vi "CRYCal Start Freq for TSR.vi"(6 "Hn":dbl=1.0, 8 "Over-samples Res.":dbl, 9 "sweep type":i32=1, 10 "FStart":dbl, 11 "Fs":dbl=2.0) -> (2 "Increment":dbl, 3 "Start Fs":dbl)   [LabVIEW 2013]
panel:
  out "x+y":dbl
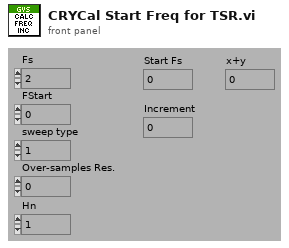
[diagram p1: front panel]
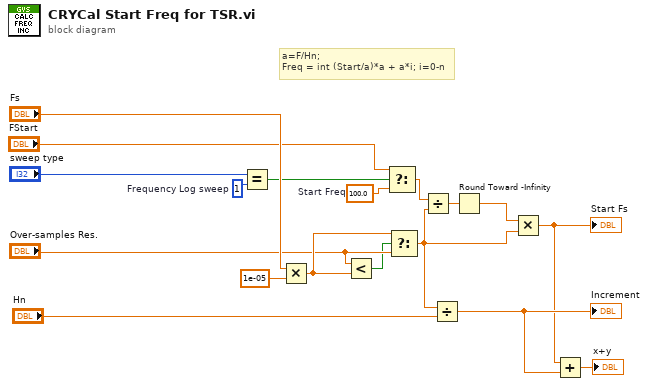
[diagram p0: block diagram]
diagram:
  w13 = 1  # Frequency Log sweep
  w15 = 100.0  # Start Freq
  # "a=F/Hn;\nFreq = int (Start/a)*a + a*i; i=0-n"
  n1 = Equal?(x="sweep type", y=w13) -> (x = y?=w11:bool)
  n2 = Multiply(x="Fs", y=1e-05) -> (x*y=w16:dbl)
  n3 = Less?(x="Over-samples Res.", y=w16) -> (x < y?=w7:bool)
  n4 = Select(t="FStart", s=w11, f=w15) -> (s? t:f=w10:dbl)
  n5 = Select(t=w16, s=w7, f="Over-samples Res.") -> (s? t:f=w1:dbl)
  n6 = Divide(x=w10, y=w1) -> (x/y=w5:dbl)
  n7 = Divide(x=w1, y="Hn") -> (x/y=w3:dbl)
  "Increment" <- w3
  n8 = Round Toward -Infinity(1:w5) -> (0:w18:dbl)
  n9 = Multiply(x=w18, y=w1) -> (x*y=w2:dbl)
  "Start Fs" <- w2
  n10 = Add(x=w2, y=w3) -> (x+y=→"x+y":dbl)
